vi "API.vi"   [LabVIEW 2024]
uses:
  atsj peakcan basic.lvlib
  get parameter - u32.vi
  set parameter - u64.vi
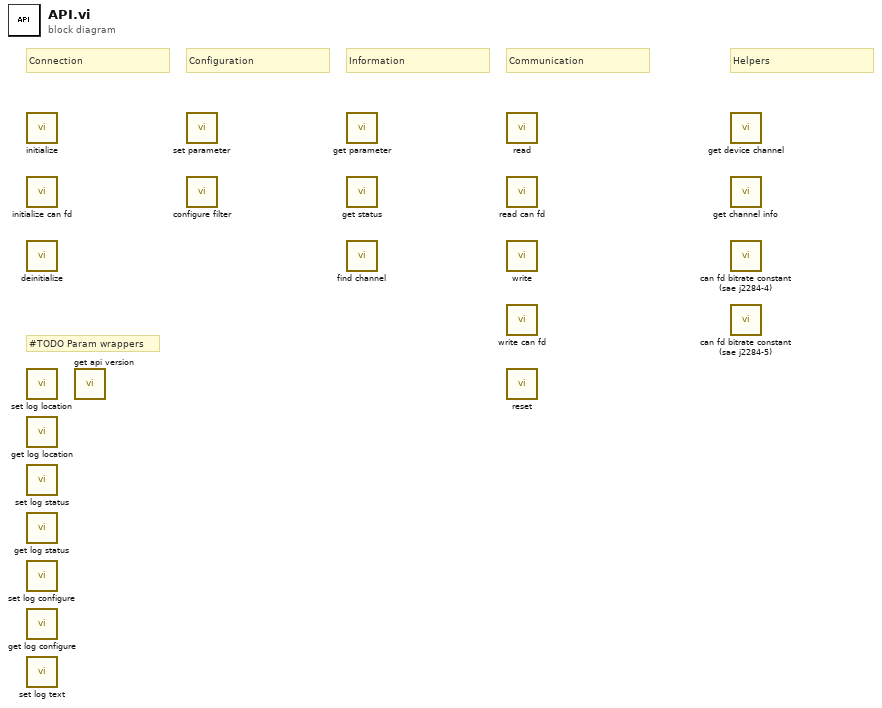
[diagram p0: block diagram]
diagram:
  # "Helpers"
  # "#TODO Param wrappers"
  # "Communication"
  # "Information"
  # "Configuration"
  # "Connection"
  n1 = call "initialize.vi"() -> ()  [unwired: 11 in, 1 out]
  n2 = call "initialize can fd.vi"() -> ()  [unwired: 11 in, 1 out]
  n3 = call "deinitialize.vi"() -> ()  [unwired: 11 in, 1 out]
  n4 = call "set log location.vi"() -> ()  [unwired: 11 in, 1 out]
  n5 = call "get log location.vi"() -> ()  [unwired: 10 in, 2 out]
  n6 = call "set log status.vi"() -> ()  [unwired: 11 in, 1 out]
  n7 = call "get log status.vi"() -> ()  [unwired: 10 in, 2 out]
  n8 = call "set log configure.vi"() -> ()  [unwired: 11 in, 1 out]
  n9 = call "get log configure.vi"() -> ()  [unwired: 9 in, 3 out]
  n10 = call "set log text.vi"() -> ()  [unwired: 11 in, 1 out]
  n11 = call "get api version.vi"() -> ()  [unwired: 10 in, 2 out]
  n12 = call-poly "set parameter.vi"() -> ()  [unwired: 11 in, 1 out]
  n13 = call "configure filter.vi"() -> ()  [unwired: 11 in, 1 out]
  n14 = call-poly "get parameter.vi"() -> ()  [unwired: 10 in, 2 out]
  n15 = call "get status.vi"() -> ()  [unwired: 10 in, 2 out]
  n16 = call "find channel.vi"() -> ()  [unwired: 10 in, 2 out]
  n17 = call "read.vi"() -> ()  [unwired: 8 in, 4 out]
  n18 = call "read can fd.vi"() -> ()  [unwired: 8 in, 4 out]
  n19 = call "write.vi"() -> ()  [unwired: 11 in, 1 out]
  n20 = call "write can fd.vi"() -> ()  [unwired: 11 in, 1 out]
  n21 = call "reset.vi"() -> ()  [unwired: 11 in, 1 out]
  n22 = call "get device channel.vi"() -> ()  [unwired: 10 in, 2 out]
  n23 = call "get channel info.vi"() -> ()  [unwired: 1 in, 1 out]
  n24 = call "can fd bitrate constant (sae j2284-4).vi"() -> ()  [unwired: 1 out]
  n25 = call "can fd bitrate constant (sae j2284-5).vi"() -> ()  [unwired: 1 out]
